vi "RoughTerrain.vi"(0 "Auto_Selection":T2=enum."None", 3 "Auto_Enable":bool, 5 "Dist_Foward":dbl=inf, 7 "Level":bool=TRUE, 9 "Encoder":dbl=-193.200372, 11 "Extra_Dist":dbl, 12 "Yaw":dbl=4.7941924449990925) -> (1 "Rough Terrain On":bool, 4 "Rest_Encoder":bool, 6 "Rest_Gyro":bool, 10 "Completed_Auto":bool, 14 "Motor Speed":dbl, 15 "Intake Arm Lowered":bool)   [LabVIEW 2015]
uses:
  Auto_Selection.ctl
  AutoEnum.ctl
  <vilib>/Rock Robotics/Network Tables/NT Read Number.vi
panel:
  in  "DB_Count":dbl=3.0
  out "Shooter_Speed":dbl=0.4
  out "Shoot":bool
  out "Stage":bool
  in  "Moat_Speed 2":dbl=-1.0 format="%#_13g"
  in  "Pamparts_Speed 2":dbl=-0.75 format="%#_13g"
  in  "Rock_Wall_Speed 2":dbl=-1.0 format="%#_13g"
  in  "Rough_Speed 2":dbl=-0.75 format="%#_13g"
  in  "Numeric 2":i32=10000
  in  "Min_Dist_Drive 2":dbl=150.0
  in  "DB_Pitch 2":dbl=4.0
  in  "Return_Enable":bool
  in  "Numeric":i32=10000
  in  "Distaince_DB":dbl=1.0
  out "error":errorcluster
  out "Enum":T1
  out "x = y?":bool
  in  "Distance Goal":dbl=180.0
  in  "Pamparts_Speed":dbl=-0.75 format="%#_13g"
  in  "Rock_Wall_Speed":dbl=-1.0 format="%#_13g"
  in  "Rough_Speed":dbl=-0.75 format="%#_13g"
  in  "Moat_Speed":dbl=-1.0 format="%#_13g"
  in  "Clear Error":bool
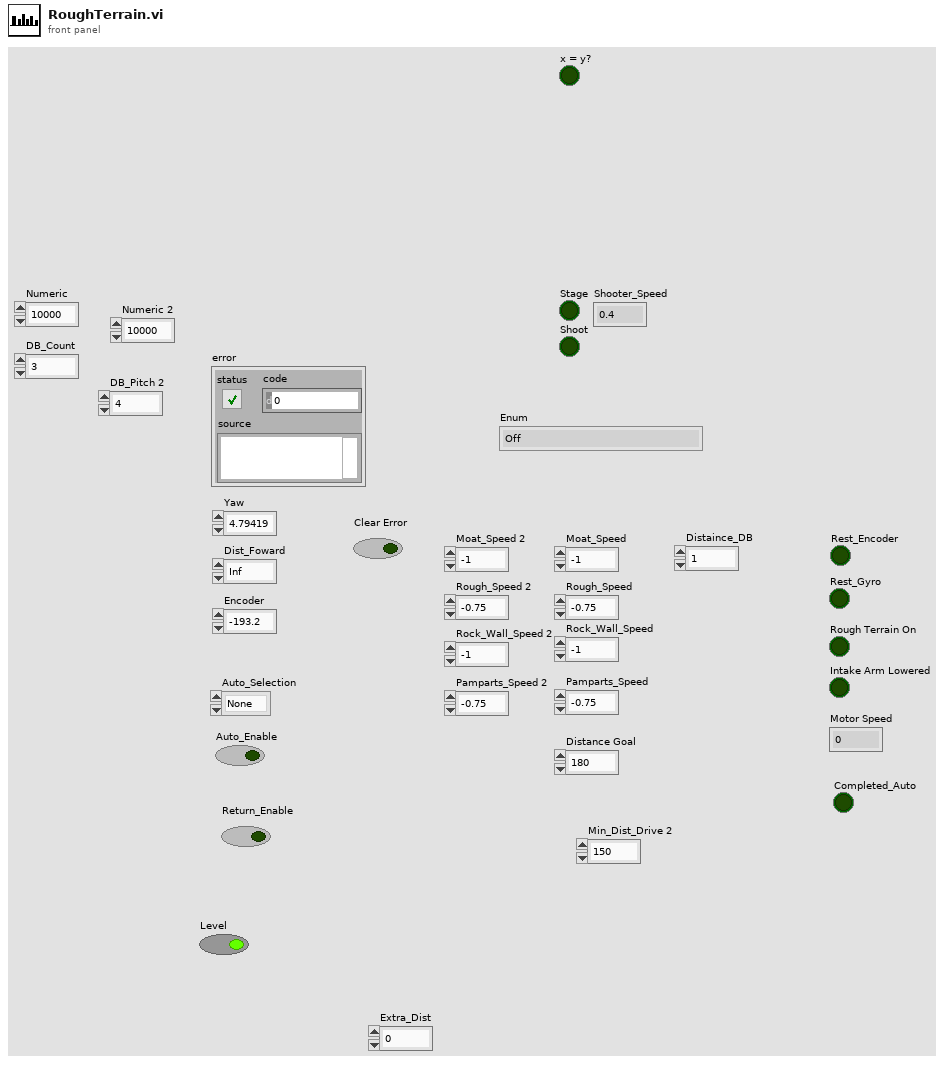
[diagram p1: front panel]
types:
  T1 = typedef "AutoEnum.ctl" = enum16{"Off", "ResetVar", "ResetOff", "BeforeTeeter", "LowerArm", "DriveForward", "Stop", "Stop One", "Drive Back", "Drive Forward Two"}
  T2 = typedef "Auto_Selection.ctl" = enum16{"Low Bar", "Rough Terrain", "Rock Wall", "Ramparts", "Moat", "Cheval de Frise", "Portcullis", "None", "One  Ball", "Shoot"}
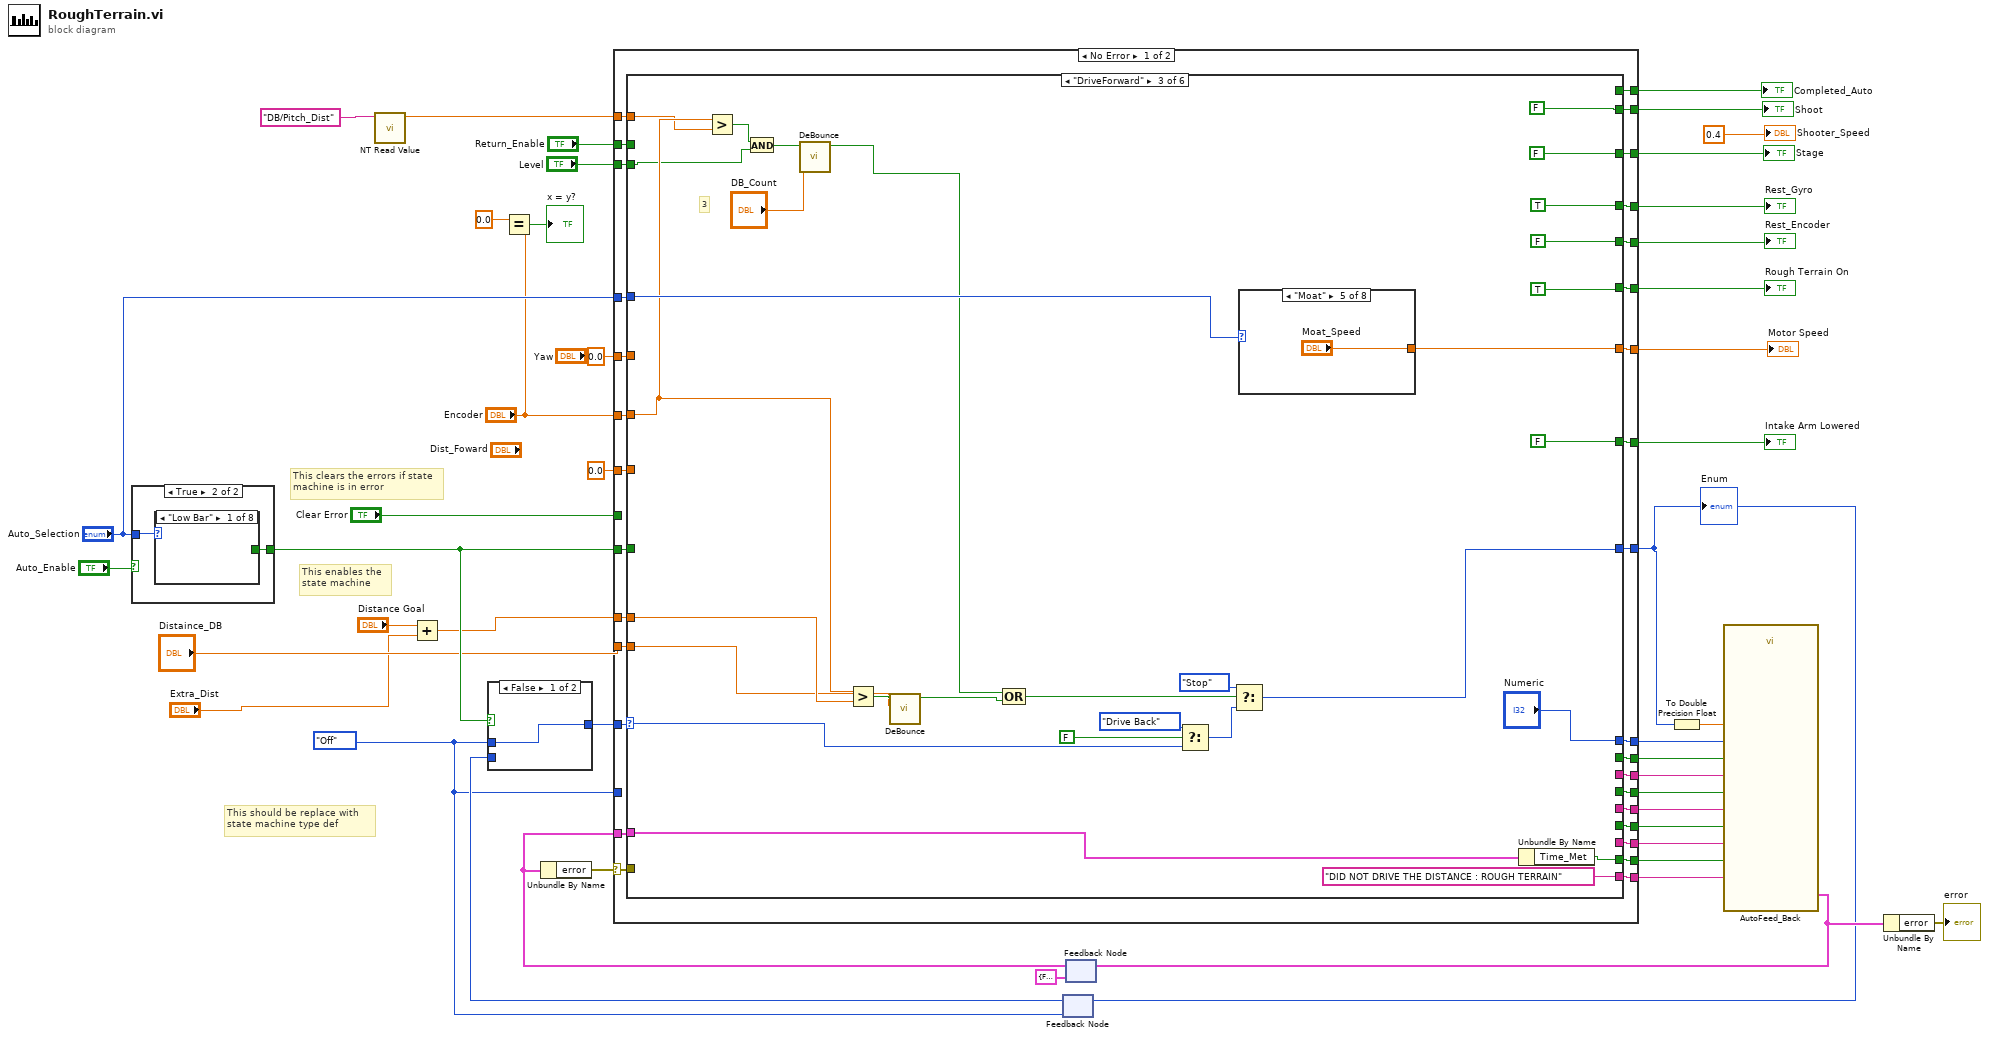
[diagram p0: block diagram]
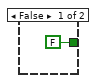
[diagram p2: hidden frame]
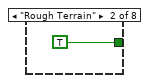
[diagram p3: hidden frame]
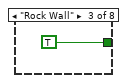
[diagram p4: hidden frame]
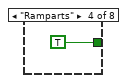
[diagram p5: hidden frame]
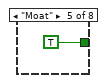
[diagram p6: hidden frame]
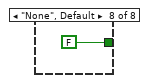
[diagram p9: hidden frame]
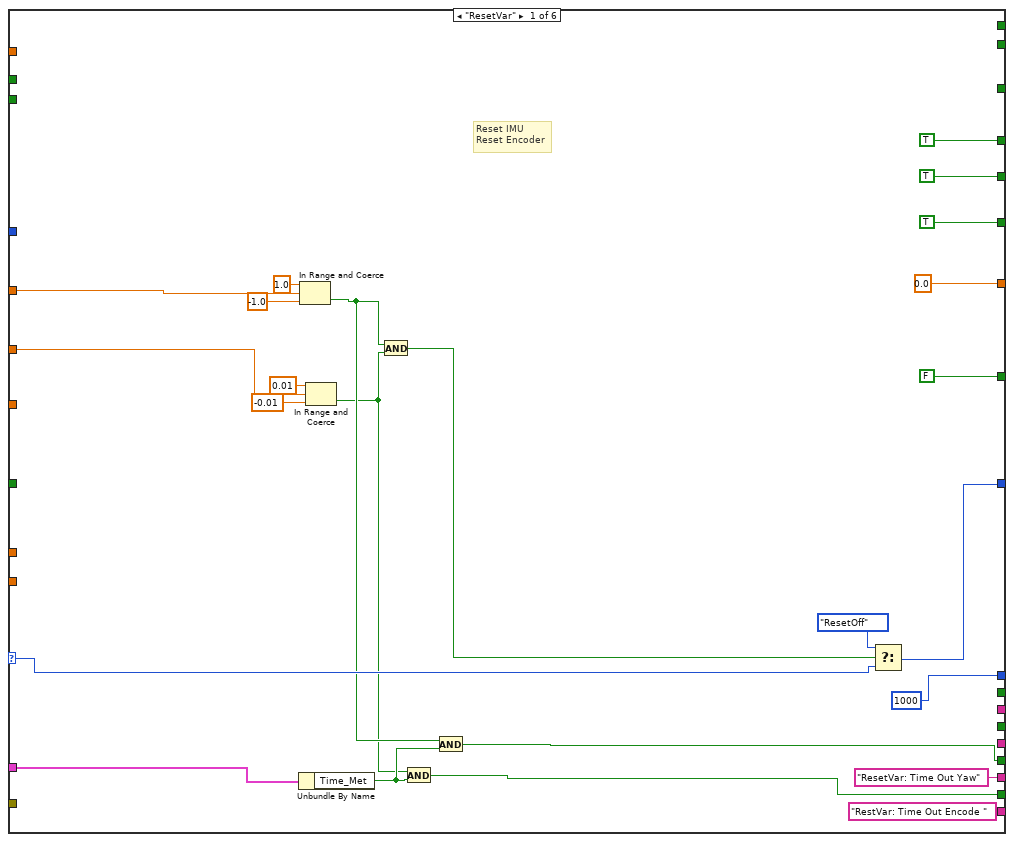
[diagram p11: hidden frame]
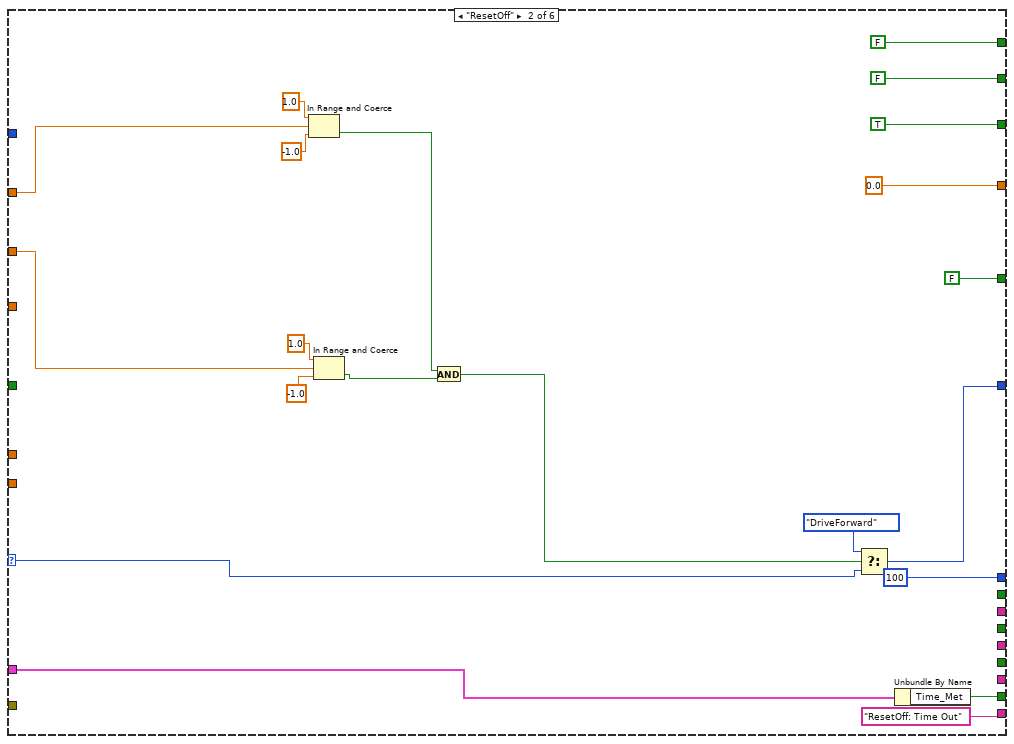
[diagram p12: hidden frame]
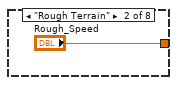
[diagram p14: hidden frame]
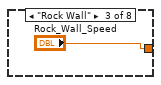
[diagram p15: hidden frame]
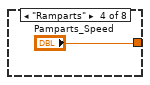
[diagram p16: hidden frame]
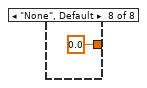
[diagram p19: hidden frame]
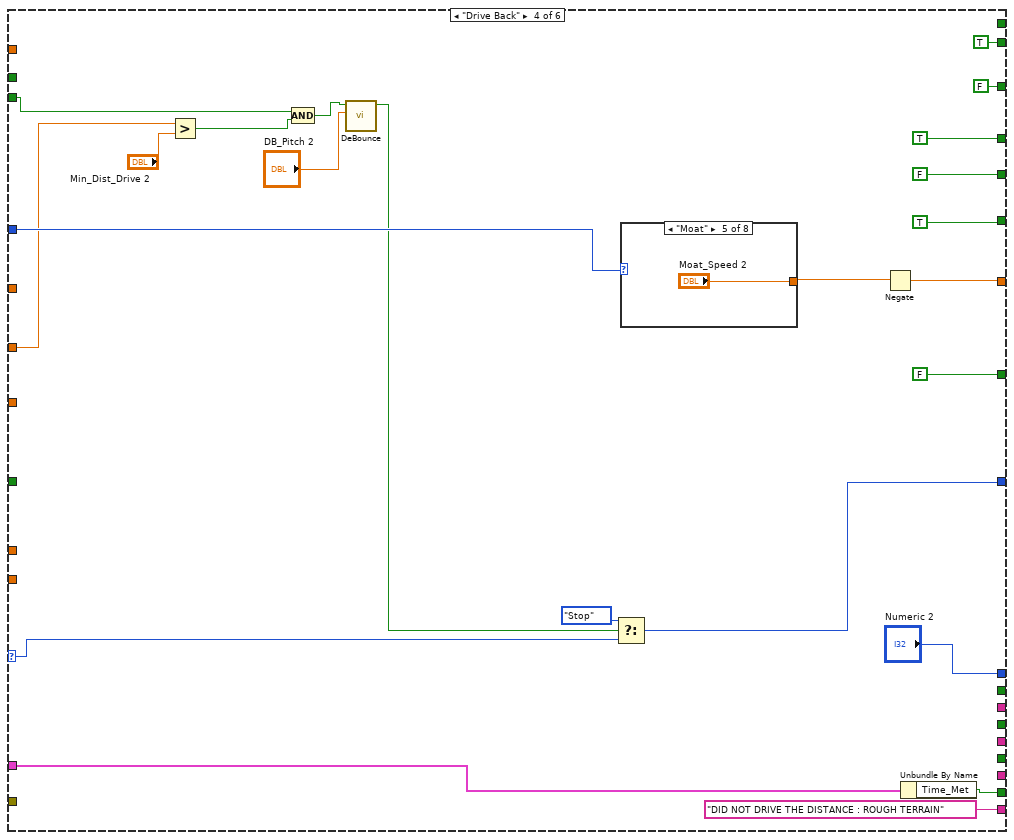
[diagram p20: hidden frame]
diagram:
  w35 = AutoEnum."Off"
  # "This clears the errors if state \nmachine is in error"
  # "This enables the \nstate machine"
  # "This should be replace with \nstate machine type def"
  n1 = case shown="True" "Auto_Enable" {
    tunnel: "Auto_Selection" -> [_ w48]
    tunnel: [FALSE w47] -> w31
    frame False {
    }
    frame True {
      n2 = case shown="\"Low Bar\"" w48 {
        tunnel: [_ TRUE TRUE TRUE TRUE _ _ FALSE] -> w47
        frame "Low Bar" {
        }
        frame "Rough Terrain" {
        }
        frame "Rock Wall" {
        }
        frame "Ramparts" {
        }
        frame "Moat" {
        }
        frame "Cheval de Frise" {
        }
        frame "Portcullis" {
        }
        frame "None", Default {
        }
      }
    }
  }
  n3 = call-poly <vilib>:"NT Read Value.vi"("Name"="DB/Pitch_Dist" ("refnum name")) -> ("Numeric"=w1:dbl)  [unwired: 9 in, 1 out]
  n4 = Add(x="Distance Goal", y="Extra_Dist") -> (x+y=w3:dbl)
  n5 = Equal?(x=0.0, y="Encoder") -> (x = y?=→"x = y?":bool)
  n6 = feedback #1(w35) -> (w37:T1)
  n7 = case shown="False" w31 {
    tunnel: w35 -> [w54 _]
    tunnel: [w54 w55] -> w38
    tunnel: w37 -> [_ w55]
    frame False {
    }
    frame True {
    }
  }
  n8 = feedback #2(cluster{"Time_Met":bool, "error ":errorcluster} {"Time_Met"=FALSE, "error "={"status"=FALSE, "code"=0, "source"=""}} ("Feedback_State")) -> (w39:cluster{"Time_Met":bool, "error ":errorcluster})
  n9 = Unbundle By Name(w39) -> ("error"=w41:errorcluster)
  n10 = case shown="No Error" w41 {
    selector: w41 -> [w81 w242]
    tunnel: [w86 FALSE] -> w45
    tunnel: [w85 FALSE] -> w44
    tunnel: [w84 w239] -> w16
    tunnel: [w83 0] -> w43
    tunnel: "Clear Error" -> [_ w241]
    tunnel: w39 -> [w82 _]
    tunnel: w31 -> [w80 _]
    tunnel: w38 -> [w79 _]
    tunnel: w35 -> [_ w239]
    tunnel: [w78 0.0] -> w34
    tunnel: [w77 FALSE] -> w33
    tunnel: [w76 FALSE] -> w32
    tunnel: 0.0 ("Yaw") -> [w75 _]
    tunnel: "Encoder" -> [w74 _]
    tunnel: 0.0 ("Dist_Foward") -> [w73 _]
    tunnel: "Auto_Selection" -> [w72 _]
    tunnel: [w71 w234] -> w28
    tunnel: [w70 FALSE] -> w27
    tunnel: [w69 FALSE] -> w26
    tunnel: [w68 FALSE] -> w25
    tunnel: [w67 w233] -> w24
    tunnel: [w66 ""] -> w23
    tunnel: [w65 ""] -> w22
    tunnel: [w64 ""] -> w21
    tunnel: w3 -> [w63 _]
    tunnel: "Level" -> [w62 _]
    tunnel: "Return_Enable" -> [w61 _]
    tunnel: [w60 FALSE] -> w10
    tunnel: [w59 FALSE] -> w9
    tunnel: [w58 FALSE] -> w7
    tunnel: "Distaince_DB" -> [w57 _]
    tunnel: w1 -> [w56 _]
    frame No Error {
      n11 = case shown="\"DriveForward\"" w79 {
        selector: w79 -> [w102 w125 w146 w170 _ w219]
        tunnel: [TRUE FALSE TRUE TRUE FALSE FALSE] -> w86
        tunnel: [TRUE FALSE FALSE FALSE FALSE FALSE] -> w85
        tunnel: [1000 100 "Numeric" "Numeric 2" 2000 0] -> w83
        tunnel: [w101 w124 w149 w180 AutoEnum."Stop" w218] -> w84
        tunnel: w82 -> [w104 w115 w150 w181 _ _]
        tunnel: w81 -> [_ _ _ _ _ _]
        tunnel: w80 -> [_ _ _ _ _ w220]
        tunnel: [0.0 0.0 w154 w174 0.0 0.0] -> w78
        tunnel: [TRUE TRUE TRUE TRUE FALSE FALSE] -> w77
        tunnel: [FALSE FALSE FALSE FALSE FALSE FALSE] -> w76
        tunnel: w75 -> [w90 w117 _ _ _ _]
        tunnel: w74 -> [w89 w116 w138 w178 _ _]
        tunnel: w73 -> [_ _ _ _ _ _]
        tunnel: w72 -> [_ _ w155 w183 _ _]
        tunnel: [_ _ _ _ _ FALSE] -> w71
        tunnel: [_ _ _ _ _ FALSE] -> w70
        tunnel: [w88 _ _ _ _ FALSE] -> w69
        tunnel: [w87 w112 w148 w179 _ FALSE] -> w68
        tunnel: [_ _ _ _ _ ""] -> w67
        tunnel: [_ _ _ _ _ ""] -> w66
        tunnel: ["ResetVar: Time Out Yaw" _ _ _ _ ""] -> w65
        tunnel: ["RestVar: Time Out Encode " ("source") "ResetOff: Time Out" ("source") "DID NOT DRIVE THE DISTANCE : ROUGH TERRAIN" ("source") "DID NOT DRIVE THE DISTANCE : ROUGH TERRAIN" ("source") _ ""] -> w64
        tunnel: w63 -> [_ _ w152 _ _ _]
        tunnel: w62 -> [_ _ w135 w168 _ _]
        tunnel: w61 -> [_ _ _ _ _ _]
        tunnel: [_ _ FALSE FALSE _ FALSE] -> w60
        tunnel: [_ _ FALSE TRUE _ FALSE] -> w59
        tunnel: [_ _ _ _ TRUE FALSE] -> w58
        tunnel: w57 -> [_ _ w141 _ _ _]
        tunnel: w56 -> [_ _ w137 _ _ _]
        frame "ResetVar" {
          # "Reset IMU\nReset Encoder"
          n12 = Unbundle By Name(w104) -> ("Time_Met"=w96:bool)
          n13 = In Range and Coerce(upper limit=1.0, x=w90, lower limit=-1.0) -> (In Range?=w95:bool)  [unwired: 1 out]
          n14 = In Range and Coerce(upper limit=0.01, x=w89, lower limit=-0.01) -> (In Range?=w91:bool)  [unwired: 1 out]
          n15 = And(x=w95, y=w91) -> (x .and. y?=w100:bool)
          n16 = And(x=w91, y=w96) -> (x .and. y?=w87:bool)
          n17 = And(x=w95, y=w96) -> (x .and. y?=w88:bool)
          n18 = Select(t=AutoEnum."ResetOff", s=w100, f=w102) -> (s? t:f=w101:T1)
        }
        frame "ResetOff" {
          n19 = In Range and Coerce(upper limit=1.0, x=w117, lower limit=-1.0) -> (In Range?=w120:bool)  [unwired: 1 out]
          n20 = In Range and Coerce(upper limit=1.0, x=w116, lower limit=-1.0) -> (In Range?=w118:bool)  [unwired: 1 out]
          n21 = And(x=w120, y=w118) -> (x .and. y?=w114:bool)
          n22 = Select(t=AutoEnum."DriveForward", s=w114, f=w125) -> (s? t:f=w124:T1)
          n23 = Unbundle By Name(w115) -> ("Time_Met"=w112:bool)
        }
        frame "DriveForward" {
          # "3"
          n24 = Greater?(x=w138, y=w137) -> (0:w136:bool)
          n25 = And(x=w136, y=w135) -> (x .and. y?=w134:bool)
          n26 = call "DeBounce.vi"("DB_Count"="DB_Count", "Value"=w134) -> ("BD_Value"=w133:bool)  [unwired: 9 in]
          n27 = Greater?(x=w138, y=w152) -> (0:w151:bool)
          n28 = call "DeBounce.vi"("DB_Count"=w141, "Value"=w151) -> ("BD_Value"=w139:bool)  [unwired: 9 in]
          n29 = Compound Arithmetic op=OR(w133, w139) -> (w140:bool)
          n30 = Select(t=AutoEnum."Drive Back", s=FALSE, f=w146) -> (s? t:f=w147:T1)
          n31 = Select(t=AutoEnum."Stop", s=w140, f=w147) -> (s? t:f=w149:T1)
          n32 = case shown="\"Moat\"" w155 {
            tunnel: [_ "Rough_Speed" "Rock_Wall_Speed" "Pamparts_Speed" "Moat_Speed" _ _ 0.0 ("Moat_Speed")] -> w154
            frame "Low Bar" {
            }
            frame "Rough Terrain" {
            }
            frame "Rock Wall" {
            }
            frame "Ramparts" {
            }
            frame "Moat" {
            }
            frame "Cheval de Frise" {
            }
            frame "Portcullis" {
            }
            frame "None", Default {
            }
          }
          n33 = Unbundle By Name(w150) -> ("Time_Met"=w148:bool)
        }
        frame "Drive Back" {
          n34 = Greater?(x=w178, y="Min_Dist_Drive 2") -> (0:w169:bool)
          n35 = Compound Arithmetic op=AND(w168, w169) -> (w167:bool)
          n36 = call "DeBounce.vi"("DB_Count"="DB_Pitch 2", "Value"=w167) -> ("BD_Value"=w171:bool)  [unwired: 9 in]
          n37 = Select(t=AutoEnum."Stop", s=w171, f=w170) -> (s? t:f=w180:T1)
          n38 = case shown="\"Moat\"" w183 {
            tunnel: [_ "Rough_Speed 2" "Rock_Wall_Speed 2" "Pamparts_Speed 2" "Moat_Speed 2" _ _ 0.0 ("Moat_Speed")] -> w175
            frame "Low Bar" {
            }
            frame "Rough Terrain" {
            }
            frame "Rock Wall" {
            }
            frame "Ramparts" {
            }
            frame "Moat" {
            }
            frame "Cheval de Frise" {
            }
            frame "Portcullis" {
            }
            frame "None", Default {
            }
          }
          n39 = Negate(x=w175) -> (-x=w174:dbl)
          n40 = Unbundle By Name(w181) -> ("Time_Met"=w179:bool)
        }
        frame "Stop" {
        }
        frame "Off", Default {
          # "Nothing : Everything Off"
          n41 = Select(t=AutoEnum."ResetVar", s=w220, f=w219) -> (s? t:f=w218:T1)
        }
      }
    }
    frame Error {
      n42 = Select(t=errorcluster {"status"=FALSE, "code"=0, "source"=""}, s=w241, f=w242) -> (s? t:f=w235:errorcluster)
      n43 = Unbundle By Name(w235) -> ("status"=w234:bool, "source"=w233:string)
    }
  }
  "Rest_Gyro" <- w45
  "Rest_Encoder" <- w44
  "Motor Speed" <- w34
  "Rough Terrain On" <- w33
  "Intake Arm Lowered" <- w32
  "Enum" <- w16
  "Stage" <- w10
  "Shoot" <- w9
  "Completed_Auto" <- w7
  n44 = feedback-in #1(w16) -> ()
  n45 = To Double Precision Float(number=w16) -> (double precision float=w36:dbl)
  n46 = call "AutoFeed_Back.vi"("Code 4"=w21, "Error_4_En"=w25, "Code 3"=w22, "Code 2"=w23, "Error_3_En"=w26, "Error_2_En"=w27, "Code 1"=w24, "Error_1_En"=w28, "Time (ms)"=w43, "State"=w36) -> ("Feedback_State"=w18:cluster{"Time_Met":bool, "error ":errorcluster})  [unwired: 1 in]
  n47 = feedback-in #2(w18) -> ()
  n48 = Unbundle By Name(w18) -> ("error"=→"error":errorcluster)
  "Shooter_Speed" <- 0.4
